vi "Configure Phase Locking.vi"(6 "Reference Clock (0: In)":u16(ring) items=["In", "Out", "Master", "Slave"], 8 "error in (no error)":errorcluster, 9 "Slave Phase Shift (0 degrees)":dbl, 10 "Phase Locking Mode (0: Independent)":u16(ring) items=["Independent", "Master", "Frequency Tracking", "Slave"], 11 "VISA resource name":refnum<visa-resource-name>) -> (0 "error out":errorcluster, 3 "VISA resource name out":refnum<visa-resource-name>)   [LabVIEW 2015, in "Fluke 28x Series.lvlib"]
doc: "Configures settings for phase-locking. Channels can be set to <b>Master</b>, <b>Slave</b>, <b>Frequency Tracking</b> or <b>Indpendent</b> operation. \n\nConnecting channels together ensures that they are controlled by another channel in the same instrument, or by another function generator through the <b>Reference Clock</b> control. \n\n<b>Note</b>: Connecting channels within the same instrument requires a multichannel instrument, i.e. Fluke 282 or Fluke 284."
uses:
  <instrlib>/Fluke 28x Series/Fluke 28x Series.lvlib
panel:
  # "Note: this control refers to the\nentire instrument"
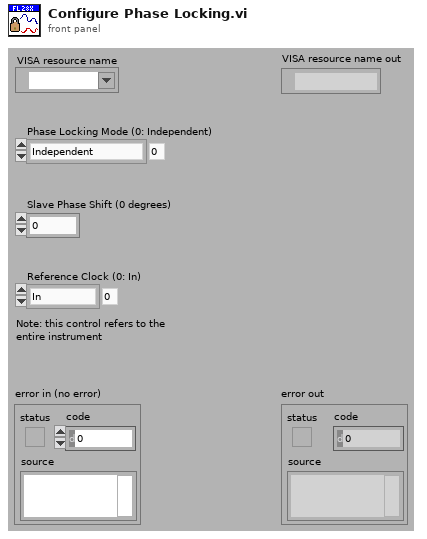
[diagram p1: front panel]
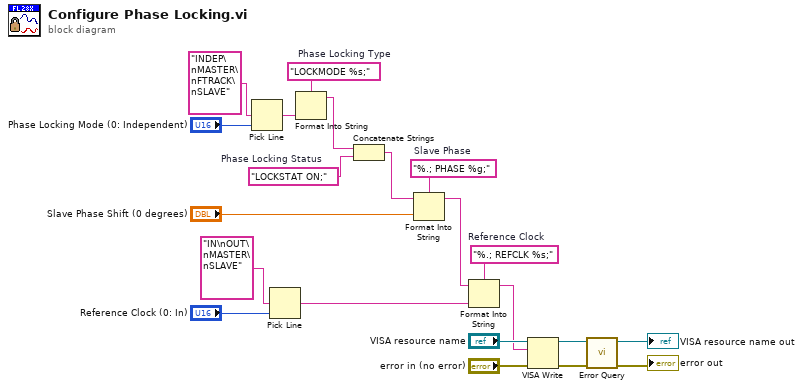
[diagram p0: block diagram]
diagram:
  w15 = "%.; REFCLK %s;"  # Reference Clock
  w19 = "%.; PHASE %g;"  # Slave Phase
  w5 = "LOCKSTAT ON;"  # Phase Locking Status
  w20 = "LOCKMODE %s;"  # Phase Locking Type
  n1 = Pick Line(multi-line string="INDEP\nMASTER\nFTRACK\nSLAVE", line index="Phase Locking Mode (0: Independent)") -> (output string=w9:string)  [unwired: 1 in]
  n2 = Pick Line(multi-line string="IN\nOUT\nMASTER\nSLAVE", line index="Reference Clock (0: In)") -> (output string=w14:string)  [unwired: 1 in]
  n3 = Format Into String(format string=w20, w9) -> (resulting string=w6:string)  [unwired: 2 in, 1 out]
  n4 = Concatenate Strings(w6, w5) -> (w4:string)
  n5 = Format Into String(format string=w19, initial string=w4, "Slave Phase Shift (0 degrees)") -> (resulting string=w13:string)  [unwired: 1 in, 1 out]
  n6 = Format Into String(format string=w15, initial string=w13, w14) -> (resulting string=w11:string)  [unwired: 1 in, 1 out]
  n7 = VISA Write(VISA resource name="VISA resource name", write buffer=w11, error in (no error)="error in (no error)") -> (VISA resource name out=w8:refnum<visa-resource-name>, error out=w7:errorcluster)  [unwired: 1 out]
  n8 = call <instrlib>:"Error Query.vi"("error in (no error)"=w7, "VISA resource name"=w8) -> ("error out"=→"error out":errorcluster, "VISA resource name out"=→"VISA resource name out":refnum<visa-resource-name>)  [unwired: 6 in, 2 out]
